vi "Tester 1.vi"() -> ()   [LabVIEW 2023, in "Error Manager.lvlib" / "Error Display Window.lvclass"]
doc: "Tester 1"
uses:
  Error Display Window.lvclass
  Error Details (cluster).ctl
  6d855587-16f8-4686-8f82-444d98388444.vi
  b33024f9-6de8-41ee-ba7d-9a2c31ef14c5.vi
  Error Display Window.lvclass/Error Display Window.ctl
panel:
  out "Error Out":errorcluster
  # "Tester 1"
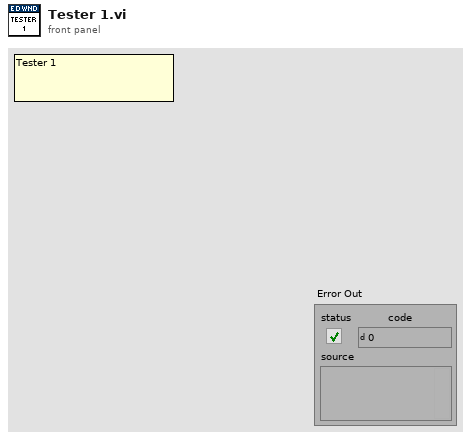
[diagram p1: front panel]
types:
  T1 = typedef "Error Manager.lvlib/Error Display Window.lvclass/Error Details (cluster).ctl" = cluster{"Error Code":i32, "Error Message":string}
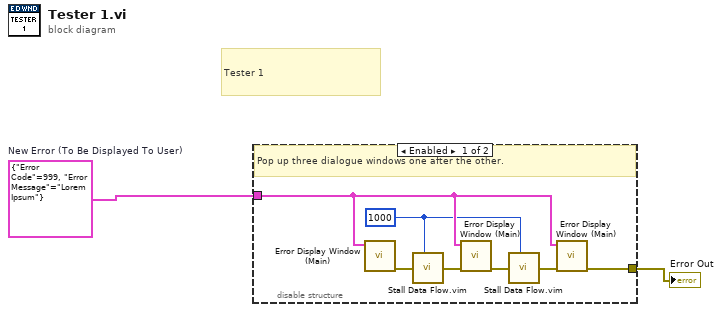
[diagram p0: block diagram]
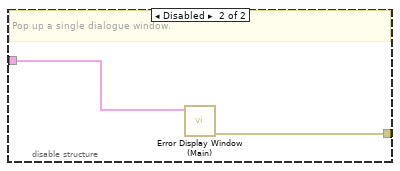
[diagram p2: hidden frame]
diagram:
  w1 = T1 {"Error Code"=999, "Error Message"="Lorem Ipsum"}  # New Error (To Be Displayed To User)
  # "Tester 1"
  n1 = disable-structure shown="Enabled" {
    disable-tunnel: [w5 w11] -> w2
    disable-tunnel: w1 -> [w4 w10]
    frame Enabled {
      w3 = u32 1000 ("milliseconds to wait")
      # "Pop up three dialogue windows one after the other."
      n2 = call "Error Display Window (Main).vi"(11:w4) -> (0:w9:errorcluster)  [unwired: 10 in]
      n3 = call "Stall Data Flow.vim"(0:w9, 1:w3) -> (3:w7:errorcluster)  [unwired: 1 out]
      n4 = call "Error Display Window (Main).vi"(8:w7, 11:w4) -> (0:w8:errorcluster)  [unwired: 9 in]
      n5 = call "Stall Data Flow.vim"(0:w8, 1:w3) -> (3:w6:errorcluster)  [unwired: 1 out]
      n6 = call "Error Display Window (Main).vi"(8:w6, 11:w4) -> (0:w5:errorcluster)  [unwired: 9 in]
    }
    frame Disabled {
      # "Pop up a single dialogue window."
      n7 = call "Error Display Window (Main).vi"(11:w10) -> (0:w11:errorcluster)  [unwired: 10 in]
    }
  }
  "Error Out" <- w2
